vi "rm.server.reserve resource.vi"(7 "notes":string, 8 "error in (no error)":errorcluster, 9 "Name in bitfile":string, 10 "Client Node Ref":T1=18446744073709551615 format="%.0x", 11 "Item Ref in":T1 format="%.0x") -> (0 "error out":errorcluster, 1 "replaced?":bool, 3 "Item Ref out":T1 format="%.0x")   [LabVIEW 2016, in "RM.Server.lvlib"]
uses:
  RM.Server.lvlib
  <vilib>/NI Veristand/Custom Device API/Custom Device Item Ref.ctl
  <vilib>/NI Veristand/Custom Device API/Set Item Property (Dependent Node Pointer).vi
  <vilib>/NI Veristand/Custom Device API/Set Item Property (String).vi
  <vilib>/NI VeriStand/Custom Device API/Custom Device API.lvlib
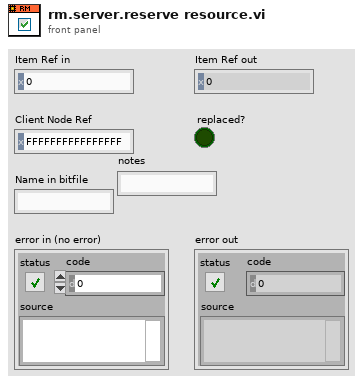
[diagram p1: front panel]
types:
  T1 = typedef "Custom Device API.lvlib/Custom Device Item Ref.ctl" = u64
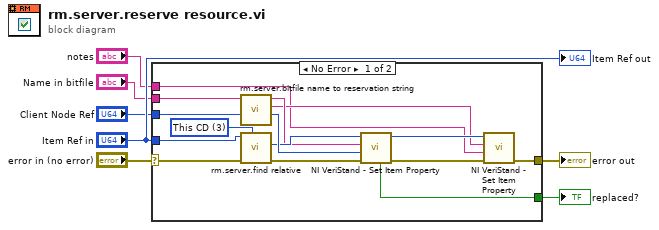
[diagram p0: block diagram]
diagram:
  n1 = case shown="No Error" "error in (no error)" {
    selector: "error in (no error)" -> [w19 w22]
    tunnel: [w10 w22] -> w6
    tunnel: "Item Ref in" -> [w17 _]
    tunnel: "Name in bitfile" -> [w14 _]
    tunnel: "Client Node Ref" -> [w21 _]
    tunnel: [w20 _] -> w2
    tunnel: "notes" -> [w8 _]
    frame No Error {
      w15 = u16 3 items=["Targets", "Controller", "Custom Devices", "This CD", "This CD/Group", "This CD/Group/SubGroup"] ("Relative Type")
      n2 = call "rm.server.bitfile name to reservation string.vi"("Name in bitfile"=w14) -> ("Notes String"=w9:string, "Reservation String"=w13:string)  [unwired: 9 in]
      n3 = call "rm.server.find relative.vi"("Relative Type"=w15, "error in (no error)"=w19, "Item Ref in"=w17) -> ("error out"=w18:errorcluster, "Relative Item Ref Out"=w16:T1)  [unwired: 4 in, 3 out]
      n4 = call-poly <vilib>:"NI VeriStand - Set Item Property.vi"("error in (no error)"=w18, "Dependent Node Ref"=w21, "Property Name"=w13, "Item Ref in"=w16) -> ("error out"=w11:errorcluster, "Item Ref out"=w12:T1, "Replaced"=w20:bool)  [unwired: 5 in]
      n5 = call-poly <vilib>:"NI VeriStand - Set Item Property.vi"("error in (no error)"=w11, "Value"=w8, "Property Name"=w9, "Item Ref in"=w12) -> ("error out"=w10:errorcluster)  [unwired: 5 in, 2 out]
    }
    frame Error {
    }
  }
  "error out" <- w6
  "replaced?" <- w2
  "Item Ref out" <- "Item Ref in"
